vi "Extract from Start and End Time.vi"(8 "Error":errorcluster, 9 "End Time":dbl, 10 "Begin Time":dbl, 11 "WavBuf":refnum<class "WavBuf.lvclass">) -> (0 "Error Out":errorcluster, 1 "Start Out":i32, 2 "Buffer Out":T1, 3 "WavBuf Out":refnum<class "WavBuf.lvclass">, 4 "End Out":i32)   [LabVIEW 2024, in "WavBuf.lvclass"]
uses:
  WavBuf.lvclass
  Universal Controls/Waveform_Data.ctl
  WavBuf.lvclass/WavBuf.ctl
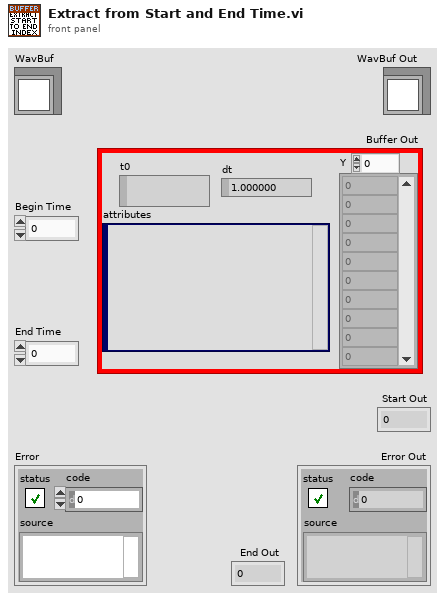
[diagram p1: front panel]
types:
  T1 = typedef "Waveform_Data.ctl" = waveform(dbl)
  T2 = typedef "Ref_DVR_Buffer.ctl" = refnum<data-value>
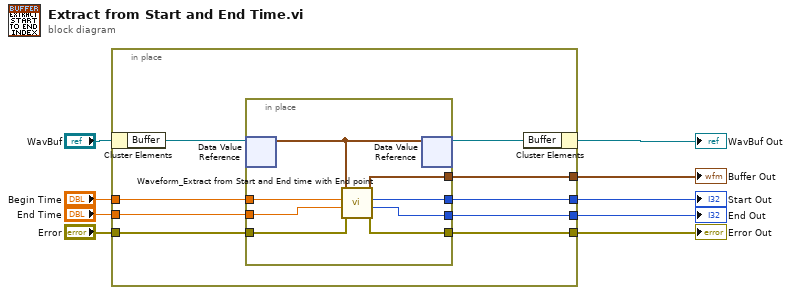
[diagram p0: block diagram]
diagram:
  n1 = in-place {
    in-place-border: "Error" -> [w18]
    in-place-border: [w17] -> w3
    in-place-border: [w16] -> w1
    in-place-border: [w15] -> w8
    in-place-border: [w14] -> w7
    in-place-border: "Begin Time" -> [w13]
    in-place-border: "End Time" -> [w12]
    n2 = in-place-cluster #1("WavBuf") -> ("Buffer"=w11:T2)
    n3 = in-place {
      in-place-border: w18 -> [w26]
      in-place-border: [w25] -> w17
      in-place-border: [w20] -> w16
      in-place-border: [w21] -> w15
      in-place-border: [w22] -> w14
      in-place-border: w13 -> [w24]
      in-place-border: w12 -> [w23]
      n4 = in-place-dvr #2(w11) -> (w19:T1)  [unwired: 1 out]
      n5 = call "Waveform_Extract from Start and End time with End point.vi"("Error"=w26, "End Time"=w23, "Begin Time"=w24, "Waveform"=w19) -> ("Error Out"=w25:errorcluster, "End Index Out"=w22:i32, "Start Index Out"=w21:i32, "Waveform Out"=w20:T1)  [unwired: 4 in]
      n6 = in-place-dvr #2(w19) -> (w10:T2)  [unwired: 1 out]
    }
    n7 = in-place-cluster #1("Buffer"=w10) -> (→"WavBuf Out":refnum<class "WavBuf.lvclass">)
  }
  "Error Out" <- w3
  "Buffer Out" <- w1
  "Start Out" <- w8
  "End Out" <- w7
